vi "Plot Properties.vi"(8 "LineTypes":sgl[](array[numeric]), 9 "LineWidths":sgl[](array[numeric]), 10 "PlotColors":sgl[](array[numeric]), 11 "XYGraph in":refnum<vi>) -> ()   [LabVIEW 2016]
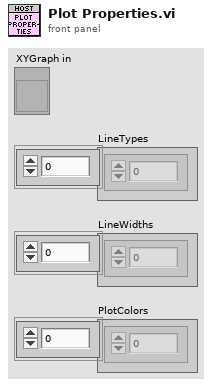
[diagram p1: front panel]
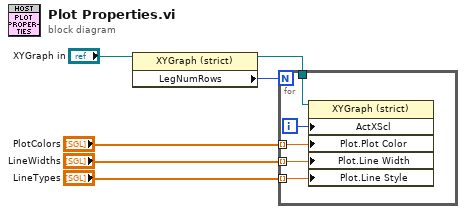
[diagram p0: block diagram]
diagram:
  n1 = property on="Property Node" class="XYGraph (strict)"(reference="XYGraph in") -> (reference out=w6:refnum<vi>, "LegNumRows"=w1:u32)  [unwired: 1 in, 1 out]
  n2 = for {
    N: w1 -> [_]
    tunnel: "PlotColors" -> [w10] mode=indexing
    tunnel: "LineWidths" -> [w9] mode=indexing
    tunnel: "LineTypes" -> [w8] mode=indexing
    tunnel: w6 -> [w7]
    i -> [w11]
    n3 = property on="Property Node" class="XYGraph (strict)"(reference=w7, "ActXScl"=w11, "Plot.Plot Color"=w10, "Plot.Line Width"=w9, "Plot.Line Style"=w8) -> ()  [unwired: 1 in, 2 out]
  }
